vi "se_sid_main.vi"(8 "se.sid.start":bool, 9 "axisXNotY":bool=TRUE, 10 "sysIdParams":T2={"sysIdOutputRate"=100, "sysIdWaveSize"=4092, "sysIdRepetitions"=50, "high"=0.0, "low"=0.0} {"sysIdOutputRate" min=10}, 11 "se.sid.i.position":T3 {"outputInt"."x" format="%.16g"; "outputInt"."y" format="%.16g"}) -> (0 "se.sid.s.repetitions":u16, 1 "se.sid.s.running":bool, 3 "se.sid.o.position":T1 {"outputInt"."x" format="%.16g"; "outputInt"."y" format="%.16g"}, 4 "se.sid.itcOutput":bool)   [LabVIEW 2016]
uses:
  <vilib>/rvi/Emulation/niFpgaEmulationIsFPGAContextNoSignature.vi
  <vilib>/rvi/Emulation/niFpgaSctlEmulationGetInTimedLoop.vi
  <vilib>/rvi/errors/niFpgaSetErrorForExecOnDevCompSimple.vi
  <vilib>/rvi/eio/common/nirviEmuReportErrorAndStop.vi
  <vilib>/rvi/DataTransferAndStorage/Container/Common/niFpgaContainerGetUniqueNameForEmu.vi
  <vilib>/rvi/FIFO/Fifo_Resource/nirvififoEmulationSetSize.vi
  <vilib>/rvi/FIFO/Fifo_Resource/nirviFifoEmulationQueueMgr.vi
  <instcachedir>/0/nirviFifoEmulationQueueMgr_E5CAEC123FF24DC58D834DCA3CDAA9B5.lvgen/nirviFifoEmulationQueueMgr_E5CAEC123FF24DC58D834DCA3CDAA9B5_010.vi
  <vilib>/rvi/FIFO/Fifo_Resource/nirvififoEmulationDetermineInputValidOut.vi
  <vilib>/rvi/FIFO/Fifo_Resource/nirvififoEmulationCreateLock.vi
  <vilib>/rvi/Emulation/niFpgaProcessEmulError.vi
  <vilib>/rvi/FIFO/Fifo_Resource/nirvififoEmulationObtainLock.vi
  <vilib>/rvi/FIFO/Fifo_Resource/nirvififoEmulationReleaseLock.vi
  <vilib>/rvi/occurrence/nirviWaitOnOccurrenceBase.vi
  <vilib>/rvi/errors/nirviReportUnexpectedCaseInternalError.vi
  <vilib>/rvi/errors/nirviReportUnexpectedCaseInternalError (U32).vi
  <vilib>/rvi/DataTransferAndStorage/Container/XNode/niFpgaContainer.xnode
  <vilib>/rvi/FIFO/Fifo_Resource/nirvififoEmulationWrite.vi
  <vilib>/eio/EIONode/EIONode.xnode
  <vilib>/rvi/eio/common/nirviEmuTemplateMethod_errors.vi
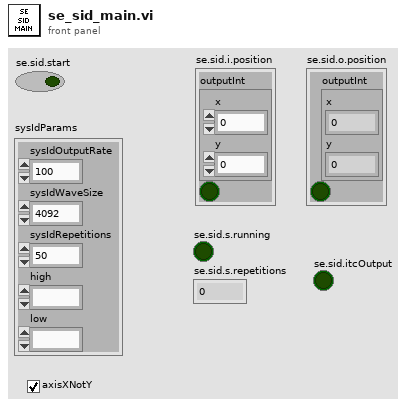
[diagram p1: front panel]
types:
  T1 = cluster{"outputInt":cluster{"sid.o.height":fxp<+/-,28,1>, "sid.o.height":fxp<+/-,28,1>}, bool}
  T2 = cluster{"sysIdOutputRate":u16, "sysIdWaveSize":u16, "sysIdRepetitions":u16, "high":fxp<+/-,17,1>, "low":fxp<+/-,17,1>}
  T3 = cluster{"outputInt":cluster{"y":fxp<+/-,16,1>, "y":fxp<+/-,16,1>}, bool}
  T4 = cluster{"sid.o.height":fxp<+/-,28,1>, "sid.o.height":fxp<+/-,28,1>}
  T5 = cluster{cluster{"sid.o.height":fxp<+/-,28,1>, "sid.o.height":fxp<+/-,28,1>}, "outputValid":bool}
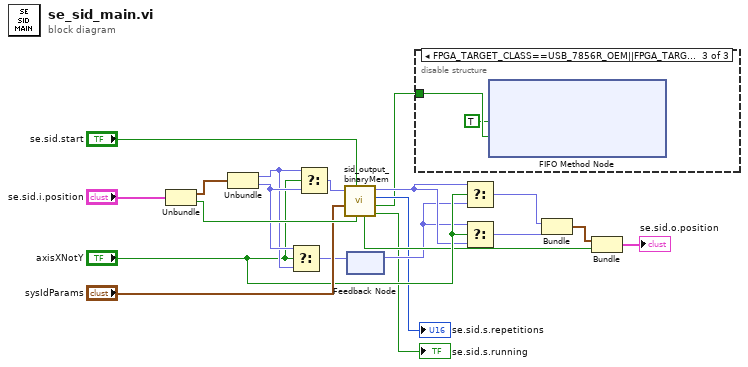
[diagram p0: block diagram]
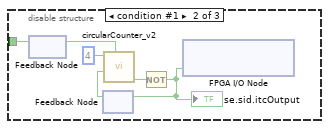
[diagram p3: hidden frame]
diagram:
  n1 = Unbundle("se.sid.i.position") -> ("outputInt"=w18:cluster{"y":fxp<+/-,16,1>, "y":fxp<+/-,16,1>}, w19:bool)
  n2 = Unbundle(w18) -> ("y"=w13:fxp<+/-,16,1>, "y"=w14:fxp<+/-,16,1>)
  n3 = Select(t=w14, s="axisXNotY", f=w13) -> (s? t:f=w10:fxp<+/-,16,1>)
  n4 = Select(t=w13, s="axisXNotY", f=w14) -> (s? t:f=w17:fxp<+/-,16,1>)
  n5 = call "sid_output_binaryMem.vi"("inputValid"=w19, "startId"="se.sid.start", "sysIdParams"="sysIdParams", "feedbackHeight"=w17) -> ("sysIdRunning"=→"se.sid.s.running":bool, "recordPoint"=w1:bool, "sysIdRep"=→"se.sid.s.repetitions":u16, "sid.o.height"=w11:fxp<+/-,28,1>, "outputValid"=w6:bool)  [unwired: 2 in, 1 out]
  n6 = feedback-in #1(w10) -> ()
  n7 = feedback #1() -> (w4:fxp<+/-,16,1>)  [unwired: 1 in]
  n8 = disable-structure shown="FPGA_TARGET_CLASS==USB_7856R_OEM||FPGA_TARGET_CLASS==USB_7856R" {
    disable-tunnel: w1 -> [_ w26 w28]
    frame condition #0 {
    }
    frame condition #1 {
      n9 = feedback-in #2(w26) -> ()
      n10 = feedback #2() -> (w21:bool)  [unwired: 1 in]
      n11 = feedback #3() -> (w23:bool)  [unwired: 1 in]
      n12 = call "circularCounter_v2.vi"("reset"=w21, "doStep"=w23, "maxCount"=u16 4) -> ("maxReached"=w24:bool)  [unwired: 5 in, 3 out]
      n13 = Not(x=w24) -> (.not. x?=w22:bool)
      "se.sid.itcOutput" <- w22
      n14 = feedback-in #3(w22) -> ()
      n15 = xnode "FPGA I/O Node"("itc.sidRecord"=w22) -> ()  [unwired: 1 in, 1 out]
    }
    frame condition #2 (active) {
      n16 = xnode ("FIFO Method Node")("Element"=TRUE, "Input Valid"=w28) -> ()  [unwired: 1 in, 2 out]
    }
  }
  n17 = Select(t=w11, s="axisXNotY", f=w4) -> (s? t:f=w9:fxp<+/-,28,1>)
  n18 = Select(t=w4, s="axisXNotY", f=w11) -> (s? t:f=w8:fxp<+/-,28,1>)
  n19 = Bundle("sid.o.height"=w9, "sid.o.height"=w8) -> (w7:T4)  [unwired: 1 in]
  n20 = Bundle(w7, "outputValid"=w6) -> (→"se.sid.o.position":T5)  [unwired: 1 in]
